vi "Test VI.vi"() -> ()   [LabVIEW 2017]
uses:
  <vilib>/Analysis/baseanly.llb/Mean (DBL).vi
  <vilib>/Analysis/NI_AALBase.lvlib
panel:
  out "mean":dbl format="%0.2f"
  out "Velocity [m/s]":i32(knob) scale=-50.0..50.0
  in  "Offset (V)":dbl
  # "Fine Adjustement"
  # "Flow Speed [m/s]"
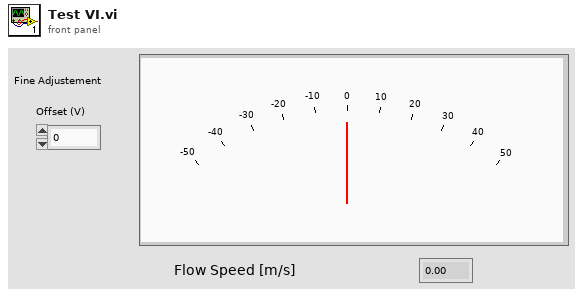
[diagram p1: front panel]
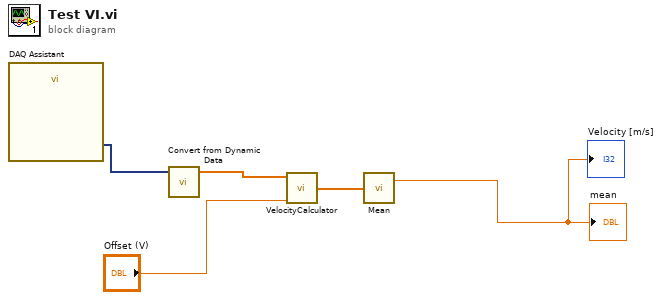
[diagram p0: block diagram]
diagram:
  n1 = call "DAQ Assistant"() -> ("data"=w2:dynamicdata)  [unwired: 17 in, 2 out]
  n2 = call "Convert from Dynamic Data"("Dynamic Data Type"=w2) -> ("Array"=w1:dbl[])  [unwired: 3 in]
  n3 = call "VelocityCalculator.vi"("Offset (V)"="Offset (V)", "Voltage Input"=w1) -> ("Veloctiy Output [m/s]"=w4:dbl[])  [unwired: 9 in]
  n4 = call-poly <vilib>:"Mean.vi"("X"=w4) -> ("mean"=→"Velocity [m/s]" →"mean":dbl)  [unwired: 1 out]
